vi "FollowPath.vi"(1 "Parameter String":string, 2 "Reinit":bool) -> (0 "Increment":bool)   [LabVIEW 2018]
uses:
  Global_Sensors.vi
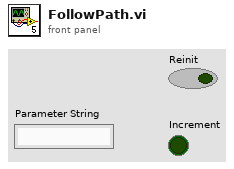
[diagram p1: front panel]
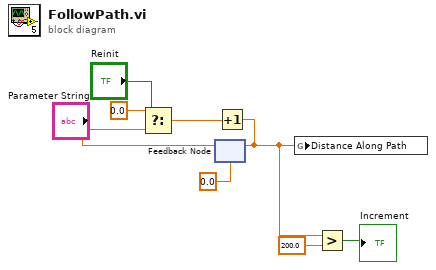
[diagram p0: block diagram]
diagram:
  n1 = feedback #1(0.0) -> (w4:dbl)
  n2 = Select(t=0.0, s="Reinit", f=w4) -> (s? t:f=w3:dbl)
  n3 = Increment(x=w3) -> (x+1=w6:dbl)
  n4 = feedback-in #1(w6) -> ()
  n5 = global write "Global_Sensors.vi" "Distance Along Path"(w6) -> ()
  n6 = Greater?(x=w6, y=200.0) -> (0:→"Increment":bool)
